vi "Log Assert Core.vi"(0 "Assert Name":string, 1 "Data Value":variant, 2 "Passed?":bool, 3 "Eval String":string, 4 "Build Timestamp":timestamp, 5 "Assert Builder":string, 6 "Default Failure Action":string, 8 "Comment":string, 10 "Assert VI UID":i32) -> ()   [LabVIEW 2016, in "AssertEngine.lvlib"]
doc: "This VI should never be directly called in an application!\n\nWill be scripted in to new assert vi's which define a specific assert instance and values to be passed to all the controls. Data Value is the only value wired to the outside world for input by the user"
uses:
  AssertEngine.lvlib
  Assert Data.ctl
  External Message Queue/Classes/Input/Input.lvclass/Input.ctl
  External Message Queue/Classes/Input/Input.lvclass
  D:/Work/Projects/Actor_Assert_API/Core/AssertEngine/External Message Queue/Classes/External Msg.lvclass
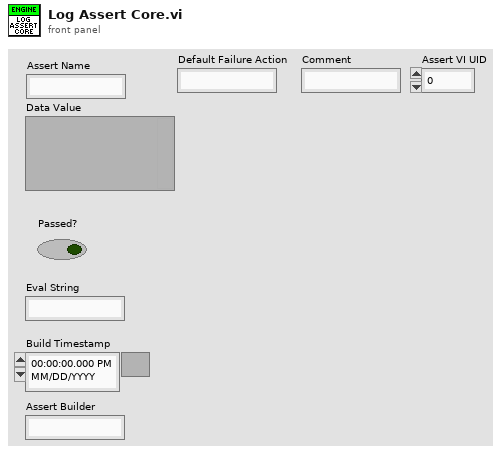
[diagram p1: front panel]
types:
  T1 = typedef "AssertEngine.lvlib/Assert Data.ctl" = cluster{"Assert Name":string, "Status":string, "Comment":string, "Eval String":string, "Failure Action":string, "Calling VI Name":string, "Assert VI Name":string, "Data Value":variant, "Assert VI UID":i32, "Assert Builder":string, "Build Timestamp":timestamp, "Last Update (Date)":string, "Top Level VI Name":string, "Data Type":string, "Last Update (Time)":string}
  T2 = typedef "Failure Action References.ctl" = cluster{"Failure Action Change Event":refnum<user-event>, "Failure Action Event Registration Refnum":refnum<event-registration>, "Assert FA SEQ":refnum<queue>}
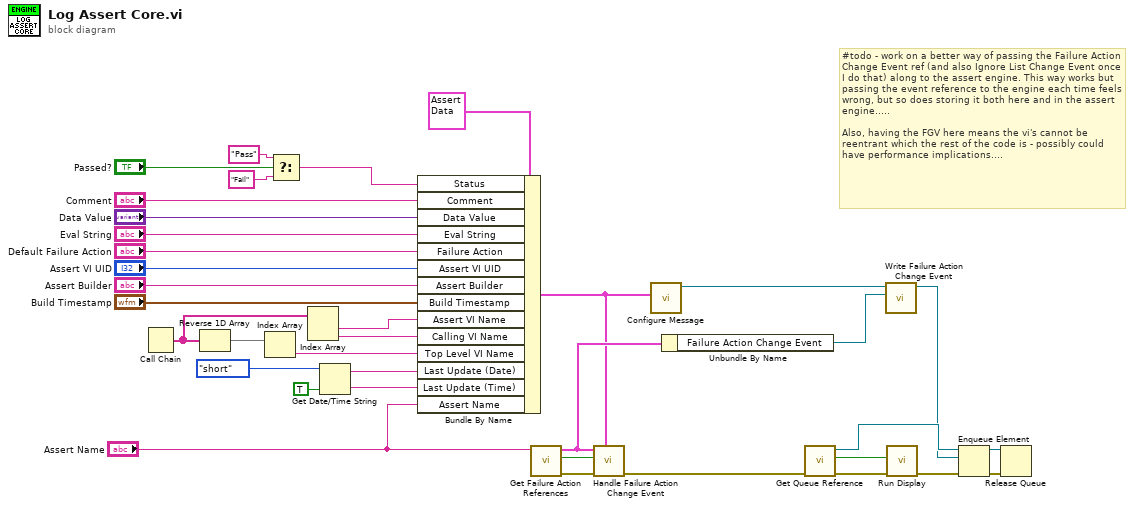
[diagram p0: block diagram]
diagram:
  # "#todo - work on a better way of passing the Failure Action Change Event ref (and also Ignore List Change Event once I do that) along to the assert engine. This way works but passing the event reference to the engine each time feels wrong, but so does storing it both here and in the assert engine.....\n\nAlso, having the FGV here means the vi's cannot be reentrant which the rest of the code is - possibly could have performance implications...."
  n1 = Call Chain() -> (call chain=w17:string[])
  n2 = Reverse 1D Array(array=w17) -> (reversed array=w16:string[])
  n3 = Index Array(array=w16) -> (element=w13:string)  [unwired: 1 in]
  n4 = Select(t="Pass", s="Passed?", f="Fail") -> (s? t:f=w23:string)
  n5 = Index Array(array=w17) -> (element #1=w15:string, element #2=w14:string)  [unwired: 2 in]
  n6 = Get Date/Time String(date format (0)=enum16{"short", "long", "abbreviated"}."short", want seconds? (F)=TRUE) -> (date string=w12:string, time string=w9:string)  [unwired: 1 in]
  n7 = Bundle By Name(cluster=T1 {"Assert Name"="", "Status"="", "Comment"="", "Eval String"="", "Failure Action"="", "Calling VI Name"="", "Assert VI Name"="", "Data Value"=variant, "Assert VI UID"=0, "Assert Builder"="", "Build Timestamp"=timestamp(0 s since 1904-01-01), "Last Update (Date)"="", "Top Level VI Name"="", "Data Type"="", "Last Update (Time)"=""} ("Assert Data"), "Status"=w23, "Comment"="Comment", "Data Value"="Data Value", "Eval String"="Eval String", "Failure Action"="Default Failure Action", "Assert VI UID"="Assert VI UID", "Assert Builder"="Assert Builder", "Build Timestamp"="Build Timestamp", "Assert VI Name"=w15, "Calling VI Name"=w14, "Top Level VI Name"=w13, "Last Update (Date)"=w12, "Last Update (Time)"=w9, "Assert Name"="Assert Name") -> (w2:T1)
  n8 = call "Get Failure Action References.vi"("Assert Name"="Assert Name") -> ("error out"=w8:errorcluster, "Created New?"=w7:bool, "Failure Action Events"=w4:T2)  [unwired: 8 in]
  n9 = call "Handle Failure Action Change Event.vi"("Assert Data"=w2, "error in (no error)"=w8, "Created New?"=w7, "Failure Action References"=w4) -> ("error out"=w6:errorcluster)  [unwired: 7 in]
  n10 = call "Configure Message.vi"("Assert Data"=w2) -> ("Input out"=w32:refnum<class "Input.lvclass">)  [unwired: 10 in]
  n11 = Unbundle By Name(w4) -> ("Failure Action Change Event"=w3:refnum<user-event>)
  n12 = call "Get Queue Reference.vi"("error in (no error)"=w6) -> ("error out"=w35:errorcluster, "created new?"=w36:bool, "Message Queue"=w33:refnum<queue>)  [unwired: 8 in]
  n13 = call "Write Failure Action Change Event.vi"("Failure Action Change Event"=w3, "Input in"=w32) -> ("Input out"=w5:refnum<class "Input.lvclass">)  [unwired: 9 in]
  n14 = call "Run Display.vi"("error in (no error)"=w35, "Run?"=w36) -> ("error out"=w31:errorcluster)  [unwired: 9 in]
  n15 = Enqueue Element(queue=w33, element=w5, error in (no error)=w31) -> (queue out=w30:refnum<queue>, error out=w29:errorcluster)  [unwired: 1 in, 1 out]
  n16 = Release Queue(queue=w30, error in (no error)=w29) -> ()  [unwired: 1 in, 3 out]
